vi "Start Measurements.vi"(6 "Reply to":refnum<class "Result Reply Msg.lvclass">, 7 "Objects enqueuers":refnum<class "Message Enqueuer.lvclass">[](array[class]), 8 "error in (no error)":errorcluster, 10 "Objects":string[](array[string]), 11 "Pulse Controller in":refnum<class "Pulse Controller.lvclass">) -> (0 "error out":errorcluster, 3 "Pulse Controller out":refnum<class "Pulse Controller.lvclass">)   [LabVIEW 2016, in "Pulse Controller.lvclass"]
uses:
  Pulse Controller.lvclass
  C:/github/LabActor/Worker/Worker.lvclass
  Template Module Messages/Result Reply Msg/Result Reply Msg.lvclass
  <vilib>/ActorFramework/Message Enqueuer/Message Enqueuer.lvclass
  Worker/Worker.lvclass/Worker.ctl
  Pulse Controller.lvclass/Pulse Controller.ctl
  Template Module/Read State.vi
  Process Controller/Process Controller.lvclass
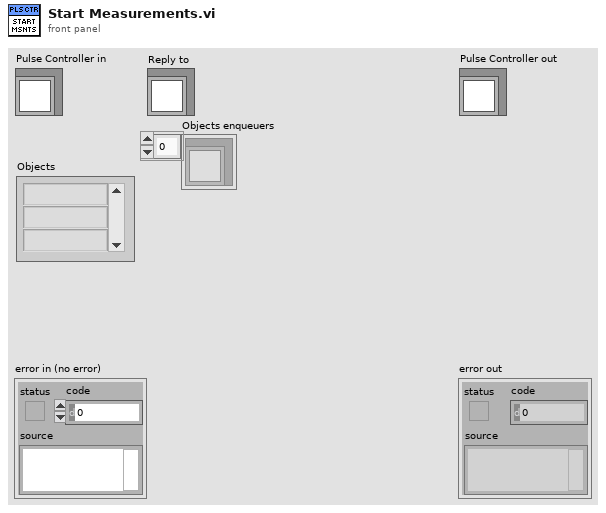
[diagram p1: front panel]
types:
  T1 = typedef "Worker State.ctl" = enum16{"Idle", "Starting", "Working", "Stopping"}
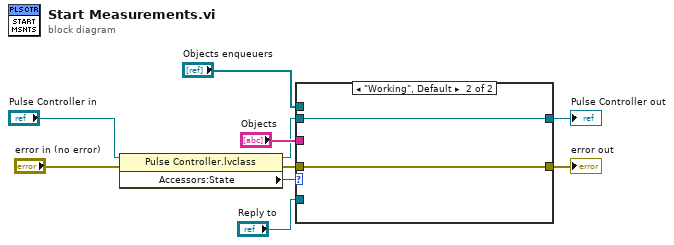
[diagram p0: block diagram]
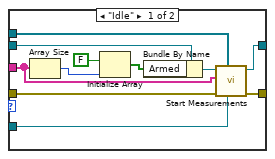
[diagram p2: hidden frame]
diagram:
  n1 = property class="Pulse Controller.lvclass"(reference="Pulse Controller in", error in="error in (no error)") -> (reference out=w3:refnum<class "Pulse Controller.lvclass">, error out=w2:errorcluster, "Accessors:State"=w4:T1)
  n2 = case shown="\"Working\", Default" w4 {
    tunnel: [w21 w23] -> w10
    tunnel: [w20 w22] -> w9
    tunnel: "Reply to" -> [w19 _]
    tunnel: "Objects enqueuers" -> [w18 _]
    tunnel: w2 -> [w17 w23]
    tunnel: "Objects" -> [w14 _]
    tunnel: w3 -> [w11 w22]
    frame "Idle" {
      n3 = Array Size(array=w14) -> (size(s)=w13:i32)
      n4 = Initialize Array(FALSE, w13) -> (w12:bool[])
      n5 = Bundle By Name(cluster=w11, "Armed"=w12) -> (w16:refnum<class "Pulse Controller.lvclass">)
      n6 = call-parent "Start Measurements.vi"("Reply to"=w19, "Objects enqueuers"=w18, "error in (no error)"=w17, "Objects"=w14, "Measure Controller in"=w16) -> ("error out"=w21:errorcluster, "Measure Controller out"=w20:refnum<class "Pulse Controller.lvclass">)  [unwired: 5 in]
    }
    frame "Working", Default {
    }
  }
  "error out" <- w10
  "Pulse Controller out" <- w9
